vi "KE622x -- Set Current Level.vi"(0 "Resource In":refnum<visa-resource-name>, 1 "Check For SCPI Errors? (T)":bool=TRUE, 7 "Current Level (A)":T1=0.1 min=-0.105 max=0.105 format="%.4p", 11 "error in (no error)":errorcluster) -> (4 "Resource Out (dupl)":refnum<visa-resource-name>, 15 "error out":errorcluster)   [LabVIEW 2013, in "Keithly user program.lvlib"]
doc: "Sets the output current level when the source is operating in a DC mode (i.e. static mode)."
uses:
  Keithly user program.lvlib
  Typedefs/KE622x -- Current Level.ctl
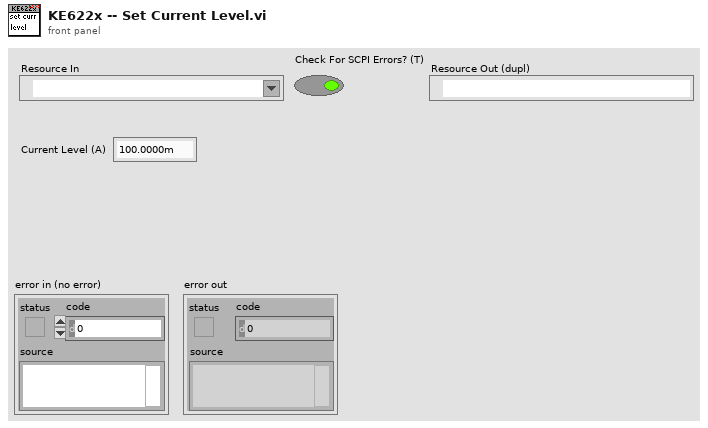
[diagram p1: front panel]
types:
  T1 = typedef "Keithly user program.lvlib/KE622x -- Current Level.ctl" = dbl
  T2 = cluster{"Auto Range?":bool, "Man / Selected\n        Range":enum16{"2nA", "20nA", "200nA", "2uA", "20uA", "200uA", "2mA", "20mA", "100mA"}}
  T3 = enum16{"2nA", "20nA", "200nA", "2uA", "20uA", "200uA", "2mA", "20mA", "100mA"}[]
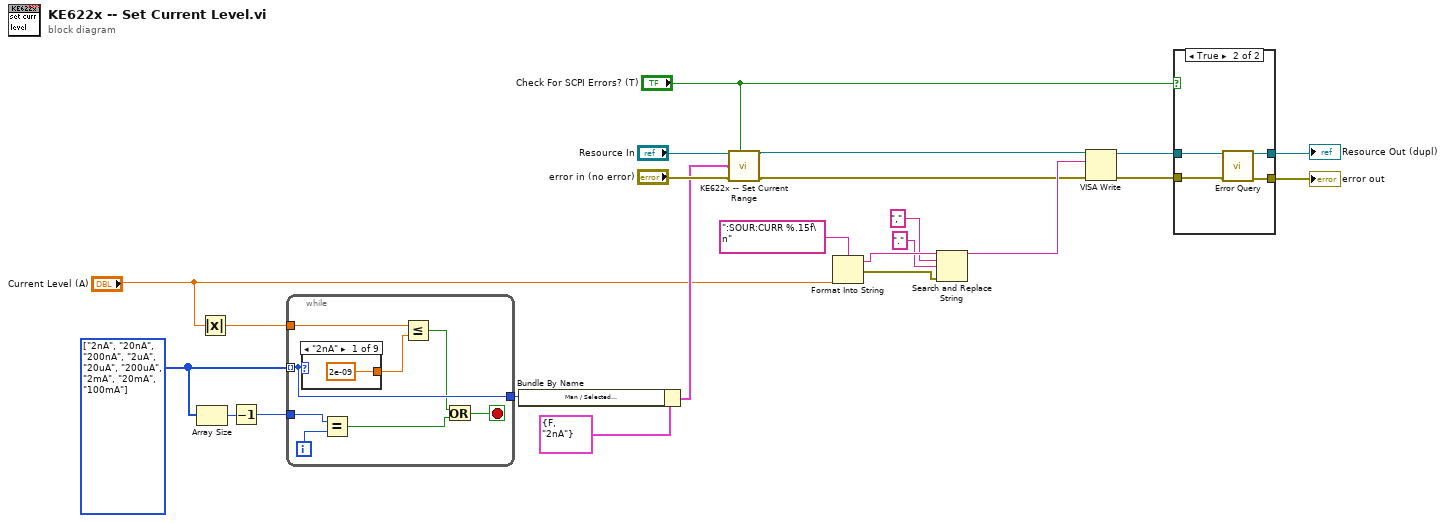
[diagram p0: block diagram]
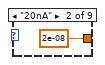
[diagram p2: hidden frame]
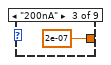
[diagram p3: hidden frame]
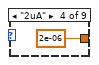
[diagram p4: hidden frame]
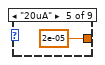
[diagram p5: hidden frame]
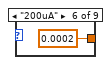
[diagram p6: hidden frame]
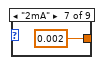
[diagram p7: hidden frame]
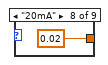
[diagram p8: hidden frame]
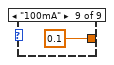
[diagram p9: hidden frame]
diagram:
  w19 = T3 [enum."2nA", enum."20nA", enum."200nA", enum."2uA", enum."20uA", enum."200uA", enum."2mA", enum."20mA", enum."100mA"] items=["2nA", "20nA", "200nA", "2uA", "20uA", "200uA", "2mA", "20mA", "100mA"]
  n1 = Array Size(array=w19) -> (size(s)=w18:i32)
  n2 = Absolute Value(x="Current Level (A)") -> (abs(x)=w20:T1)
  n3 = Decrement(x=w18) -> (x-1=w17:i32)
  n4 = while {
    tunnel: w20 -> [w31]
    tunnel: w19 -> [w30] mode=indexing
    tunnel: [w30] -> w16
    tunnel: w17 -> [w26]
    i -> [w27]
    stop <- w25 stop-if-true
    n5 = case shown="\"2nA\"" w30 {
      tunnel: [2e-09 2e-08 2e-07 2e-06 2e-05 0.0002 0.002 0.02 0.1] -> w29
      frame "2nA" {
      }
      frame "20nA" {
      }
      frame "200nA" {
      }
      frame "2uA" {
      }
      frame "20uA" {
      }
      frame "200uA" {
      }
      frame "2mA" {
      }
      frame "20mA" {
      }
      frame "100mA" {
      }
    }
    n6 = Equal?(x=w26, y=w27) -> (x = y?=w24:bool)
    n7 = Less Or Equal?(x=w31, y=w29) -> (x <= y?=w28:bool)
    n8 = Or(x=w28, y=w24) -> (x .or. y?=w25:bool)
  }
  n9 = Bundle By Name(cluster=T2 {"Auto Range?"=FALSE, "Man / Selected\n        Range"=enum."2nA"} ("Current Range"), "Man / Selected\n        Range"=w16) -> (w2:T2)
  n10 = call "KE622x -- Set Current Range.vi"("Resource In"="Resource In", "Check For SCPI Errors? (T)"="Check For SCPI Errors? (T)", "Current Range"=w2, "error in (no error)"="error in (no error)") -> ("Resource Out (dupl)"=w6:refnum<visa-resource-name>, "error out"=w3:errorcluster)  [unwired: 10 in]
  n11 = Format Into String(format string=":SOUR:CURR %.15f\n", "Current Level (A)") -> (resulting string=w12:string, error out=w11:errorcluster)  [unwired: 2 in]
  n12 = Search and Replace String(input string=w12, search string=",", replace string="." ("replace string (\"\")"), error in=w11) -> (result string=w8:string)  [unwired: 4 in, 3 out]
  n13 = VISA Write(VISA resource name=w6, write buffer=w8, error in (no error)=w3) -> (VISA resource name out=w22:refnum<visa-resource-name>, error out=w21:errorcluster)  [unwired: 1 out]
  n14 = case shown="True" "Check For SCPI Errors? (T)" {
    tunnel: w22 -> [w42 w46]
    tunnel: w21 -> [w41 w44]
    tunnel: [w41 w43] -> w13
    tunnel: [w42 w45] -> w14
    frame False {
    }
    frame True {
      n15 = call "Error Query.vi"("VISA Resource In"=w46, "error in (no error)"=w44) -> ("VISA Resource Out (dupl)"=w45:refnum<visa-resource-name>, "error out"=w43:errorcluster)  [unwired: 10 in, 2 out]
    }
  }
  "Resource Out (dupl)" <- w14
  "error out" <- w13
